vi "in_is increasing.vi"(11 "X":dbl[](array[numeric])) -> (2 "is increasing":bool, 3 "X dup":dbl[](array[numeric]))   [LabVIEW 2017, in "NI_Gmath.lvlib"]
uses:
  NI_Gmath.lvlib
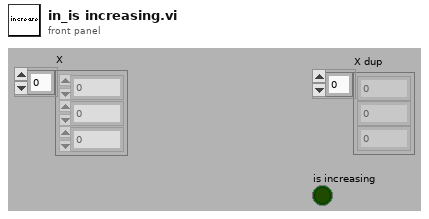
[diagram p1: front panel]
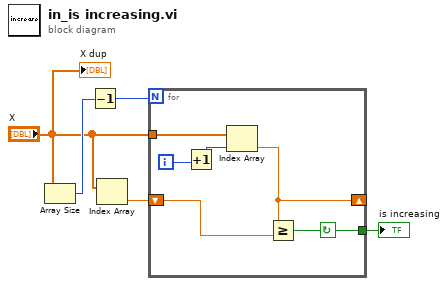
[diagram p0: block diagram]
diagram:
  n1 = Array Size(array="X") -> (size(s)=w4:i32)
  n2 = Decrement(x=w4) -> (x-1=w5:i32)
  n3 = Index Array(array="X") -> (element=w3:dbl)  [unwired: 1 in]
  n4 = for {
    N: w5 -> [_]
    tunnel: "X" -> [w11]
    shift-right: [w8] -> _
    shift-left: w3 -> [w7]
    tunnel: [w6] -> w1
    i -> [w10]
    stop <- w6 continue-if-true
    n5 = Increment(x=w10) -> (x+1=w9:i32)
    n6 = Index Array(array=w11, index=w9) -> (element=w8:dbl)
    n7 = Greater Or Equal?(x=w8, y=w7) -> (x >= y?=w6:bool)
  }
  "is increasing" <- w1
  "X dup" <- "X"
